vi "GEN2_Ping.vi"(8 "error in (no error)":errorcluster, 10 "ID":u8, 11 "VISA Refnum in":refnum<visa-resource-name>) -> (0 "error out":errorcluster, 1 "ERROR":u8, 2 "Version":T1 {"DRV Ver" format="%x"; "HW Ver" format="%x"; "FW Ver" format="%x"}, 3 "VISA Refnum out":refnum<visa-resource-name>)   [LabVIEW 2016, in "GEN_2.lvlib"]
uses:
  GEN_2.lvlib
  GEN2_Instructions.ctl
  <vilib>/ErrorRing/Error Ring.xnode
  <vilib>/Utility/error.llb/Error Cluster From Error Code.vi
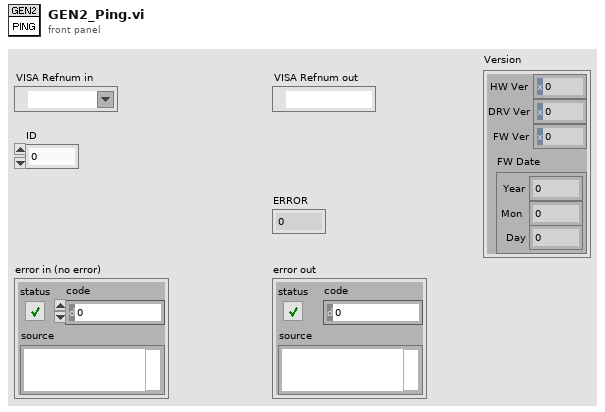
[diagram p1: front panel]
types:
  T1 = cluster{"HW Ver":u8, "DRV Ver":u8, "FW Ver":u16, "FW Date":cluster{"Year":u32, "Mon":u32, "Day":u32}}
  T2 = enum16{"big-endian, network order", "native, host order", "little-endian"}
  T3 = typedef "GEN_2.lvlib/GEN2_Instructions.ctl" = u8
  T4 = cluster{"ID":u8, "ERROR":u8, "ChechSumError?":bool, "Data":string}
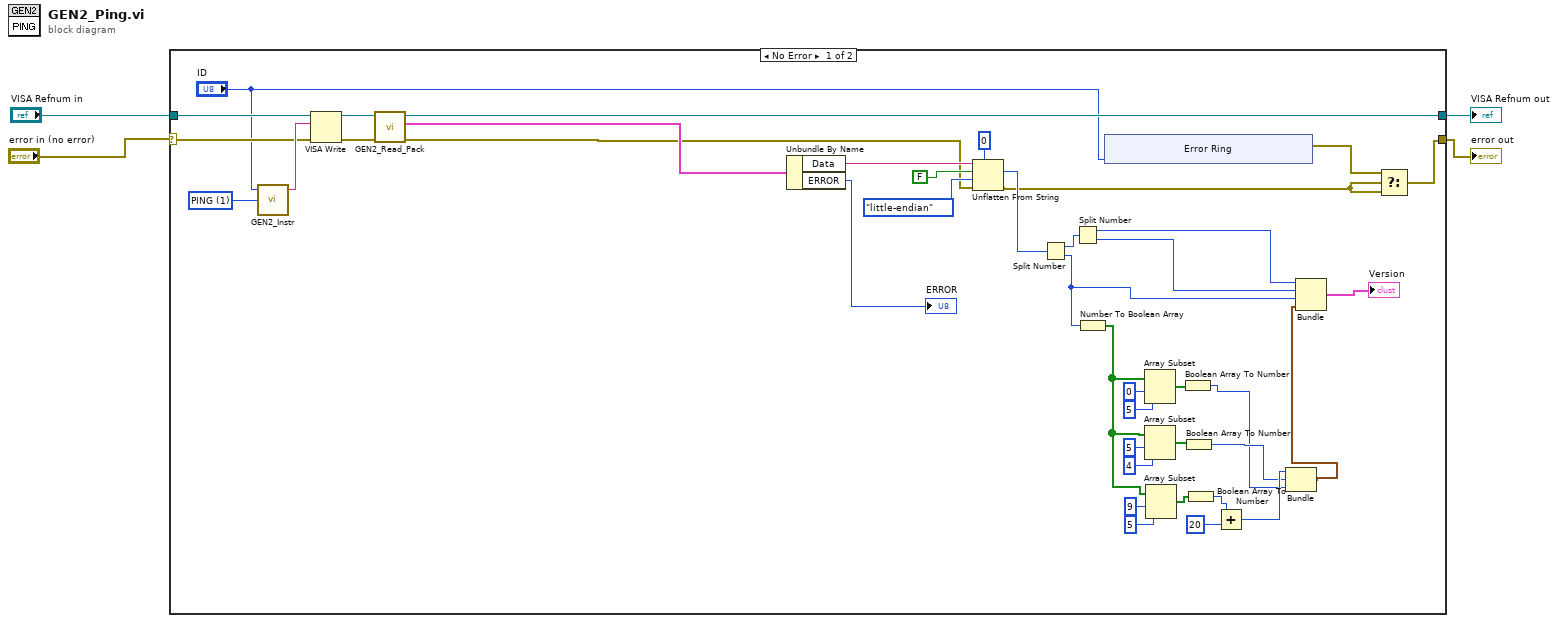
[diagram p0: block diagram]
diagram:
  n1 = case shown="No Error" "error in (no error)" {
    selector: "error in (no error)" -> [w33 w53]
    tunnel: [w39 w52] -> w4
    tunnel: [w5 w53] -> w3
    tunnel: "VISA Refnum in" -> [w34 w52]
    frame No Error {
      w40 = T3 1 items=["PING"=1, "READ_STAT"=2, "WRITE_STAT"=3, "READ_CONFIG"=4, "WRITE_CONFIG"=5, "SAVE_CONFIG"=6] ("Instruction")
      n2 = call "GEN2_Instr.vi"("Instruction"=w40, "ID"="ID") -> ("Output"=w35:string)  [unwired: 3 in]
      n3 = VISA Write(VISA resource name=w34, write buffer=w35, error in (no error)=w33) -> (VISA resource name out=w37:refnum<visa-resource-name>, error out=w38:errorcluster)  [unwired: 1 out]
      n4 = call "GEN2_Read_Pack.vi"("error in (no error)"=w38, "VISA Refnum in"=w37) -> ("error out"=w7:errorcluster, "Pack data"=w36:T4, "VISA Refnum out"=w39:refnum<visa-resource-name>)  [unwired: 7 in]
      n5 = Unbundle By Name(w36) -> ("Data"=w44:string, "ERROR"=→"ERROR":u8)
      n6 = Unflatten From String(type=u32 0, binary string=w44, data includes array or string size? (T)=FALSE, byte order (0:big-endian, network order)=T2."little-endian", error in (no error)=w7) -> (value=w32:u32, error out=w6:errorcluster)  [unwired: 1 out]
      n7 = Split Number(x=w32) -> (hi(x)=w31:u16, lo(x)=w11:u16)
      n8 = Split Number(x=w31) -> (hi(x)=w13:u8, lo(x)=w12:u8)
      n9 = Number To Boolean Array(number=w11) -> (Boolean array=w23:bool[])
      n10 = xnode "Error Ring"("parameter 0"="ID") -> ("error out"=w8:errorcluster)
      n11 = Array Subset(array=w23, index=0, length=5) -> (w22:bool[])
      n12 = Array Subset(array=w23, index=5, length=4) -> (w21:bool[])
      n13 = Array Subset(array=w23, index=9, length=5) -> (w20:bool[])
      n14 = Boolean Array To Number(Boolean array=w22) -> (number=w15:u32)
      n15 = Boolean Array To Number(Boolean array=w21) -> (number=w16:u32)
      n16 = Boolean Array To Number(Boolean array=w20) -> (number=w19:u32)
      n17 = Add(x=w19, y=u32 20) -> (x+y=w17:u32)
      n18 = Bundle(w17, w16, w15) -> (w10:cluster{u32, u32, u32})  [unwired: 1 in]
      n19 = Bundle(w13, w12, w11, w10) -> (→"Version":cluster{u8, u8, u16, cluster{u32, u32, u32}})  [unwired: 1 in]
      n20 = Select(t=w8, s=w6, f=w6) -> (s? t:f=w5:errorcluster)
    }
    frame Error {
    }
  }
  "VISA Refnum out" <- w4
  "error out" <- w3
